vi "rasterScanning.vi"() -> ()   [LabVIEW 2017]
uses:
  <vilib>/rvi/Emulation/niFpgaSctlEmulationGetInTimedLoop.vi
  <vilib>/rvi/Emulation/niFpgaProcessEmulError.vi
  <vilib>/rvi/Emulation/niFpgaGetClockAttributes.vi
  <vilib>/rvi/Emulation/niFpgaEmulationReportErrorSimple.vi
  <vilib>/rvi/eio/common/nirviEmuTemplateMethod_errors.vi
  <vilib>/rvi/Emulation/niFpgaCriticalErrorInLSC.vi
  <vilib>/rvi/interface/RandomDataEmulation/niFpgaRandomDataHandleErrors.vi
  <vilib>/eio/EIONode/EIONode.xnode
  <vilib>/rvi/DataTransferAndStorage/Container/XNode/niFpgaContainer.xnode
  <vilib>/rvi/interface/RandomDataEmulation/nirviRandomDataFpgaReadWriteTemplate.vi
panel:
  in  "y threshold":fxp<+/-,20,5>=0.0050048828125
  in  "x threshold":fxp<+/-,20,5>=0.0050048828125
  out "SettleCheckBuffer":u16=25
  out "a tor buffer":fxp<+,17,1>[](array[numeric])=[1.9999847412109375, 1.9999847412109375, 1.9999847412109375, 1.9999847412109375, 1.9999847412109375, 1.9999847412109375, 1.9999847412109375, 1.9999847412109375, 1.9999847412109375, 1.9999847412109375, 1.9999847412109375, 1.9999847412109375, 1.9999847412109375, 1.9999847412109375, 1.9999847412109375, 1.9999847412109375, 1.9999847412109375, 1.9999847412109375, 1.9999847412109375, 1.9999847412109375, 1.9999847412109375, 1.9999847412109375, 1.9999847412109375, 1.9999847412109375, 1.9999847412109375]
  out "b tor buffer":fxp<+,17,1>[](array[numeric])=[1.9999847412109375, 1.9999847412109375, 1.9999847412109375, 1.9999847412109375, 1.9999847412109375, 1.9999847412109375, 1.9999847412109375, 1.9999847412109375, 1.9999847412109375, 1.9999847412109375, 1.9999847412109375, 1.9999847412109375, 1.9999847412109375, 1.9999847412109375, 1.9999847412109375, 1.9999847412109375, 1.9999847412109375, 1.9999847412109375, 1.9999847412109375, 1.9999847412109375, 1.9999847412109375, 1.9999847412109375, 1.9999847412109375, 1.9999847412109375, 1.9999847412109375]
  in  "Stage Clock (uSec)":fxp<+,32,32>=500.0
  in  "deflection threshold":fxp<+/-,20,5>=0.0050048828125
  in  "z threshold":fxp<+/-,20,5>=0.0050048828125
  out "stageIndicator":u8=1
  in  "Scan Clock (uSec)":fxp<+,32,32>=10.0
  out "increment_y_move":fxp<+/-,55,5>=0.01171875
  out "increment_x_move":fxp<+/-,55,5>=0.01171875
  out "increment_x":fxp<+/-,55,5>=0.01171875
  out "x_pos_final":fxp<+/-,50,5>=0.005859375
  out "y_pos_final":fxp<+/-,50,5>=0.005859375
  in  "ImageToSample":T1={"image size_x"=256, "image size_y"=256, "sample start_x"=0.0, "sample start_y"=0.0, "sample end_x"=3.0, "sample end_y"=3.0}
  out "line counter":u16
  out "end line signal":bool
  in  "pixel segment":u32
  in  "deflection control":T2={"SetPoint (V)"=0.0, "scanning I"=0.03125, "scanning P"=0.0498046875, "Initial I (V)"=0.0, "Upper Limit (V)"=8.0, "Lower Limit (V)"=-8.0}
  out "deflection sensor":fxp<+/-,20,5>=-0.271331787109375
  out "zControlMode":bool
  in  "z control":T3={"SetPoint (V)"=-0.19999980926513672, "I"=0.03125, "P"=0.0498046875, "Initial I (V)"=0.0, "Upper Limit (V)"=8.0, "Lower Limit (V)"=-8.0}
  in  "Z Clock (uSec)":fxp<+,32,32>=10.0
  out "signalToRecord":bool
  out "z output":fxp<+/-,64,29>=-3.5890110712498426
  in  "Sampling Clock (uSec)":fxp<+,32,32>=1500.0
  in  "XY Clock (uSec)":fxp<+,32,32>=50.0
  out "y output":fxp<+/-,64,29>=0.29396580904722214
  out "x output":fxp<+/-,64,29>=0.00029289722442626953
  out "x sensor":fxp<+/-,20,5>
  out "y sensor":fxp<+/-,20,5>=-0.285125732421875
  in  "y control":T2={"SetPoint (V)"=0.0, "scanning I"=0.03125, "scanning P"=0.0498046875, "Initial I (V)"=0.0, "Upper Limit (V)"=8.0, "Lower Limit (V)"=-8.0}
  in  "x control":T2={"SetPoint (V)"=0.0, "scanning I"=0.03125, "scanning P"=0.0498046875, "Initial I (V)"=0.0, "Upper Limit (V)"=8.0, "Lower Limit (V)"=-8.0}
  out "signalToStop":bool
  out "x_pos":fxp<+/-,50,5>=0.005859375
  out "y_pos":fxp<+/-,50,5>=0.005859375
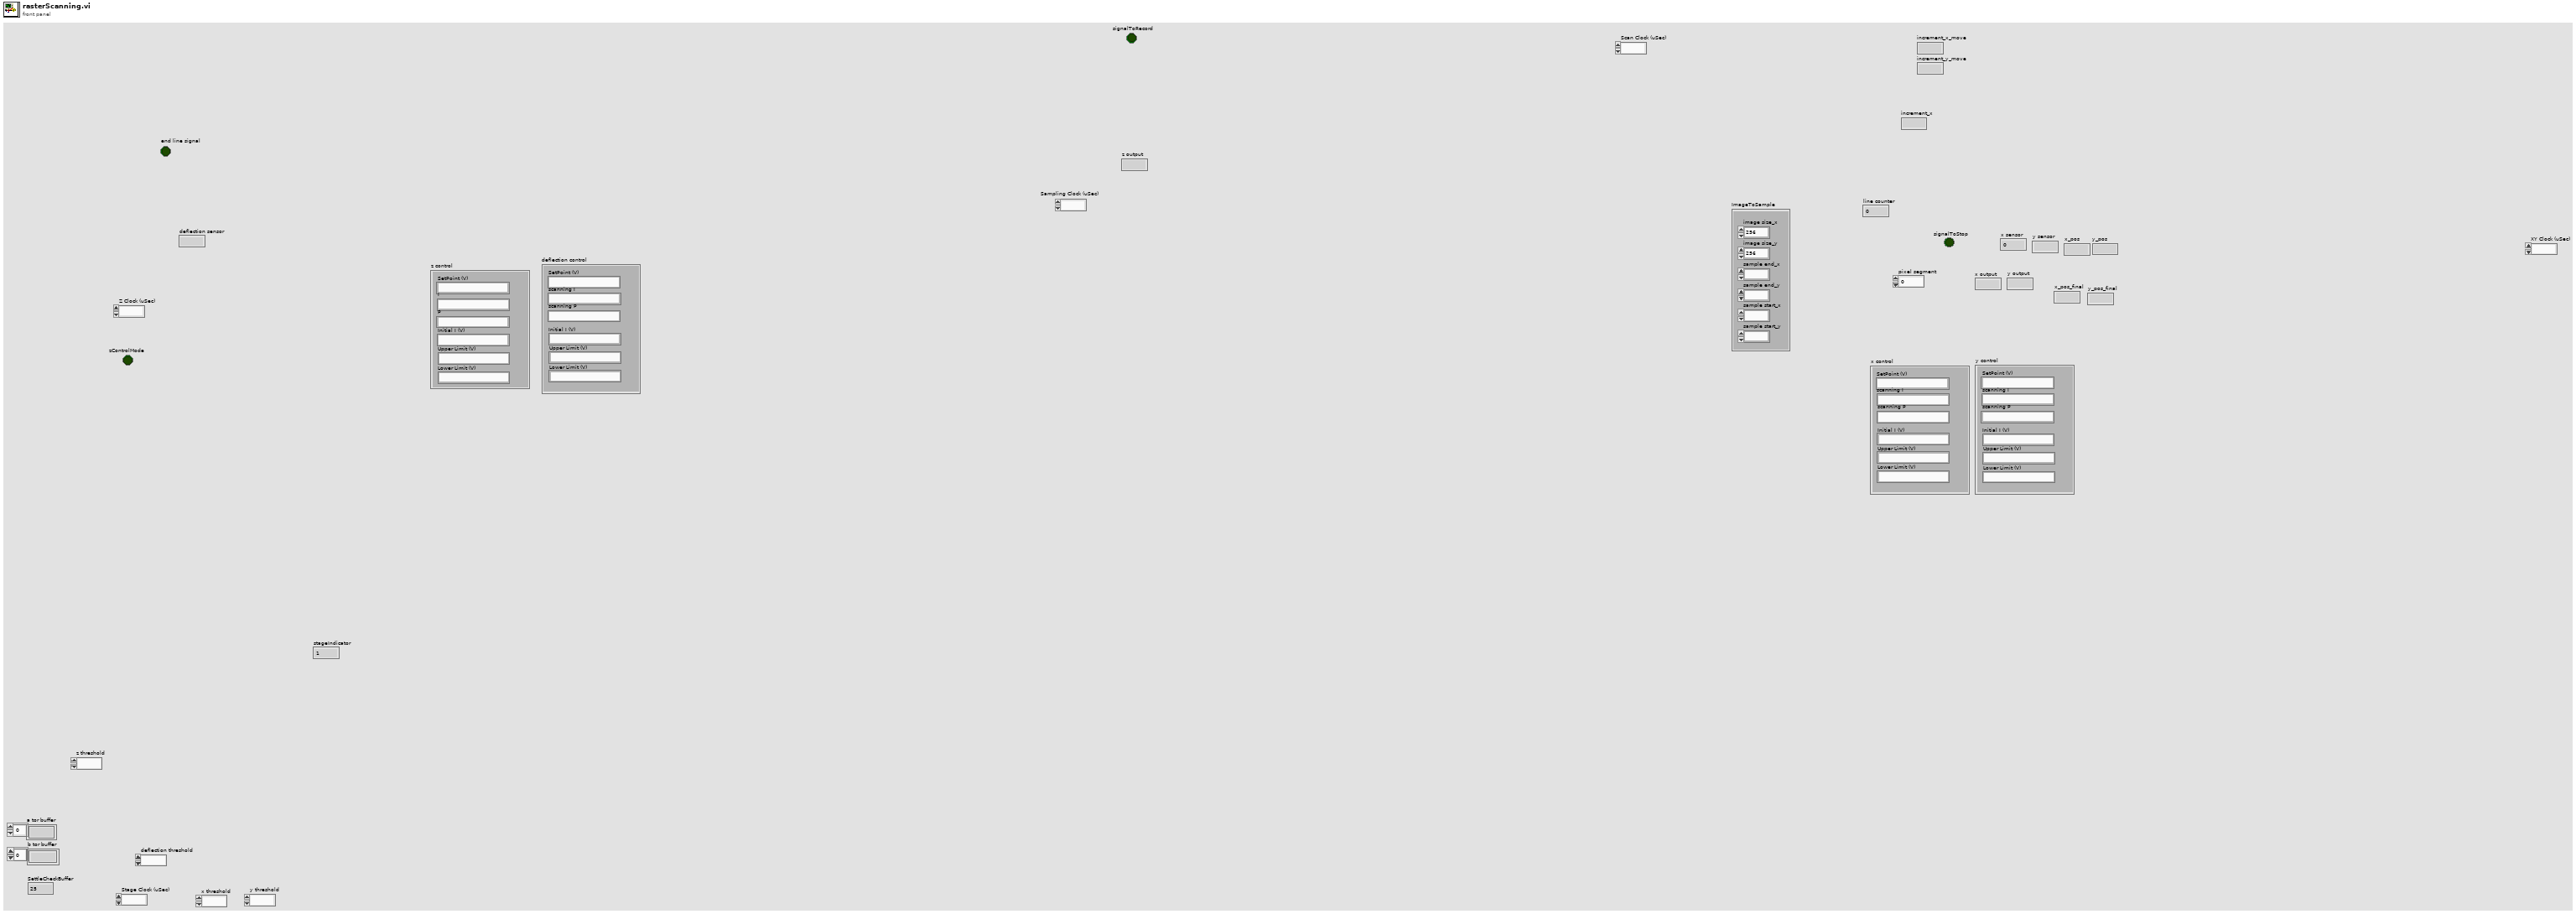
[diagram p1: front panel]
types:
  T1 = cluster{"image size_x":u16, "image size_y":u16, "sample start_x":fxp<+/-,26,5>, "sample start_y":fxp<+/-,26,5>, "sample end_x":fxp<+/-,26,5>, "sample end_y":fxp<+/-,26,5>}
  T2 = cluster{"SetPoint (V)":fxp<+/-,26,5>, "scanning I":fxp<+,21,13>, "scanning P":fxp<+,15,5>, "Initial I (V)":fxp<+/-,10,5>, "Upper Limit (V)":fxp<+/-,26,5>, "Lower Limit (V)":fxp<+/-,26,5>}
  T3 = cluster{"SetPoint (V)":fxp<+/-,26,5>, "I":fxp<+,21,13>, "P":fxp<+,15,5>, "Initial I (V)":fxp<+/-,10,5>, "Upper Limit (V)":fxp<+/-,26,5>, "Lower Limit (V)":fxp<+/-,26,5>}
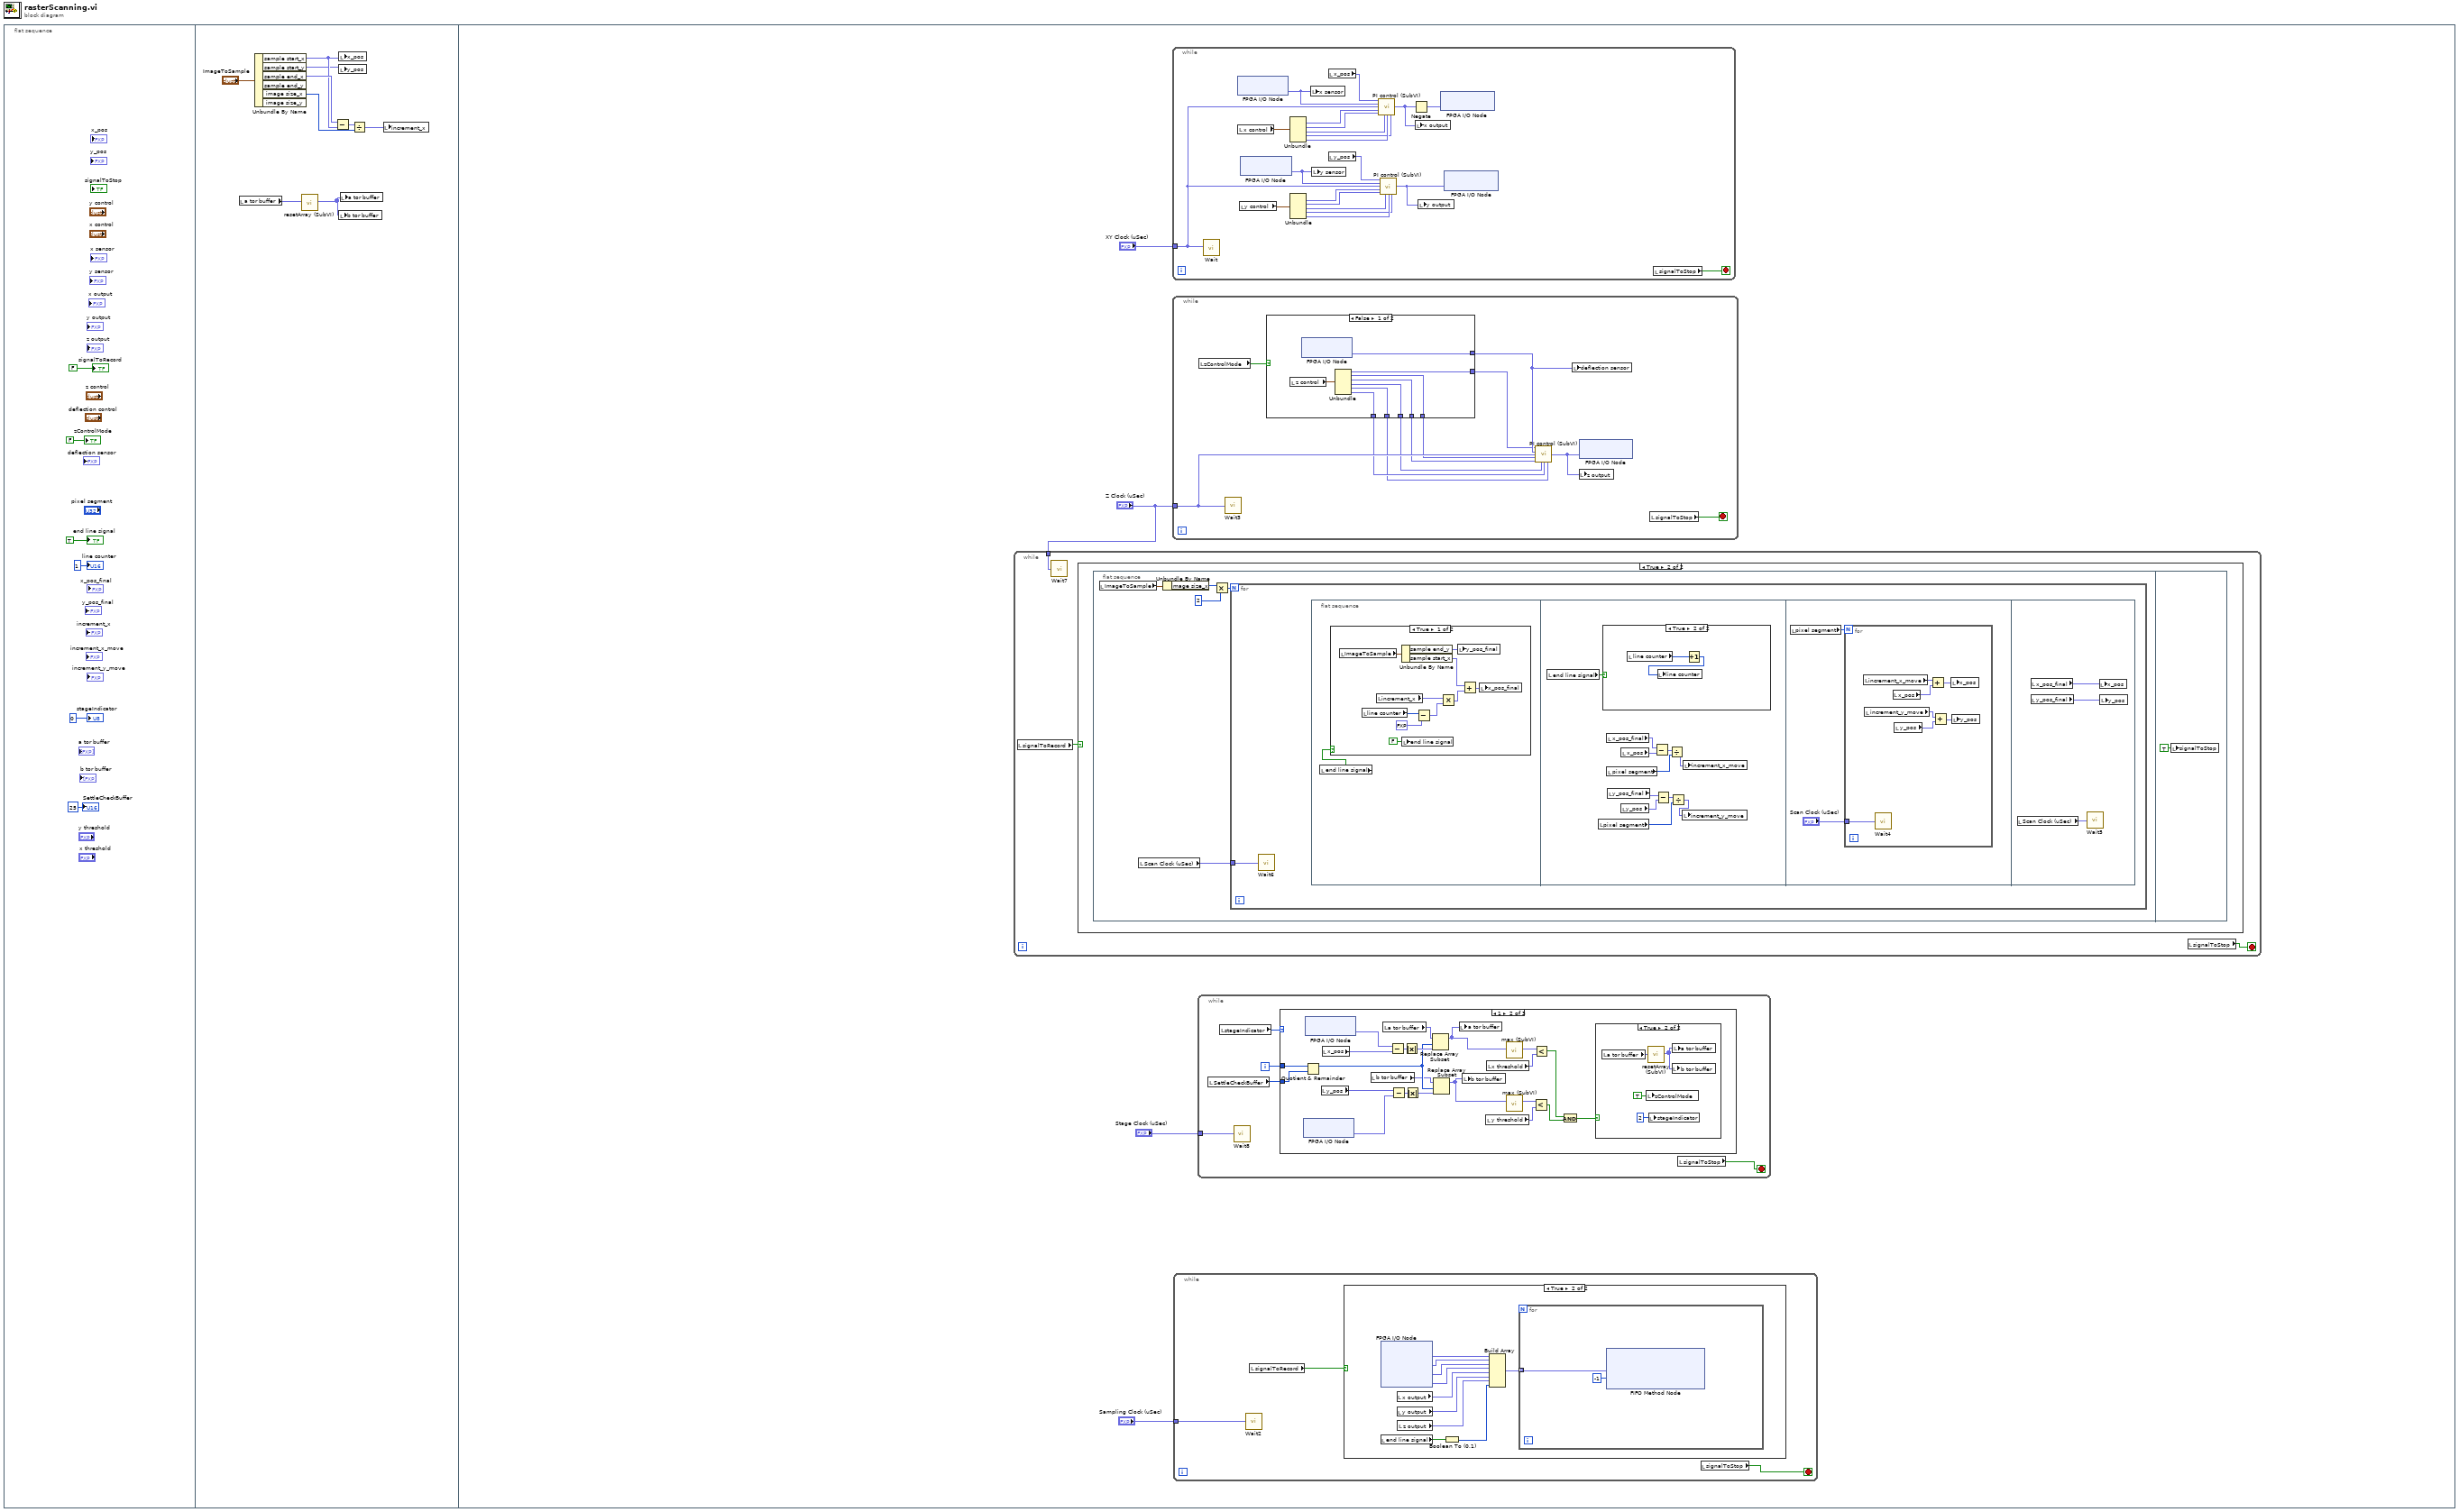
[diagram p0: block diagram]
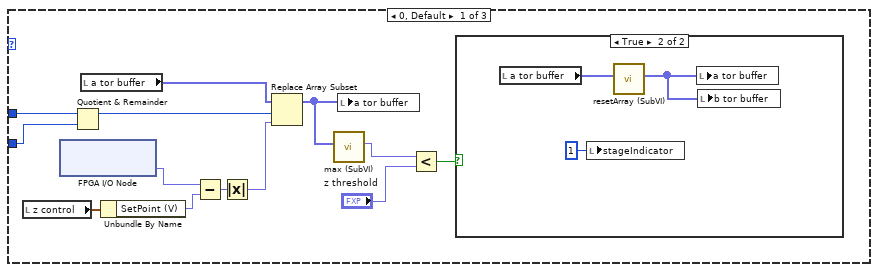
[diagram p2: hidden frame]
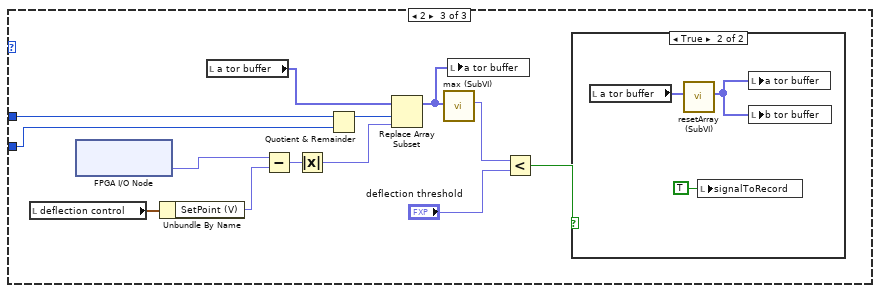
[diagram p5: hidden frame]
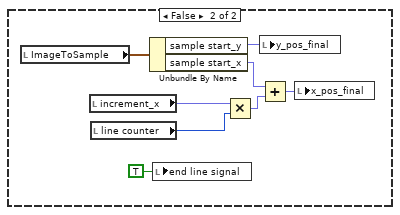
[diagram p8: hidden frame]
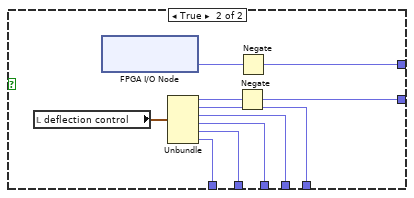
[diagram p10: hidden frame]
diagram:
  n1 = flat-sequence {
    frame #0 {
      "signalToRecord" <- FALSE ("signalToRecord")
      "zControlMode" <- FALSE ("zControlMode")
      "end line signal" <- TRUE ("end line signal")
      "line counter" <- u16 1 ("line counter")
      "stageIndicator" <- u8 0 ("stageIndicator")
      "SettleCheckBuffer" <- u16 25 ("SettleCheckBuffer")
    }
    frame #1 {
      n2 = local read "a tor buffer"() -> (w8:fxp<+,17,1>[])
      n3 = Unbundle By Name("ImageToSample") -> ("sample start_x"=w13:fxp<+/-,26,5>, "sample start_y"=w11:fxp<+/-,26,5>, "sample end_x"=w14:fxp<+/-,26,5>, "image size_x"=w10:u16)  [unwired: 2 out]
      n4 = call "resetArray (SubVI).vi"("a samples in"=w8) -> ("a samples out"=w7:fxp<+/-,64,32>[])  [unwired: 10 in]
      n5 = Subtract(x=w14, y=w13) -> (x-y=w12:fxp<+/-,27,6>)
      n6 = local write "x_pos"(w13) -> ()
      n7 = local write "y_pos"(w11) -> ()
      n8 = local write "b tor buffer"(w7) -> ()
      n9 = local write "a tor buffer"(w7) -> ()
      n10 = Divide(x=w12, y=w10) -> (x/y=w9:fxp<+/-,43,6>)
      n11 = local write "increment_x"(w9) -> ()
    }
    frame #2 {
      n12 = while {
        tunnel: "Z Clock (uSec)" -> [w84]
        stop <- w85 stop-if-true
        n13 = local read "signalToRecord"() -> (w83:bool)
        n14 = call "Wait7"("Count(uSec)"=w84) -> ()  [unwired: 1 out]
        n15 = case shown="True" w83 {
          frame False {
          }
          frame True {
            n16 = flat-sequence {
              frame #0 {
                n17 = local read "ImageToSample"() -> (w90:T1)
                n18 = local read "Scan Clock (uSec)"() -> (w86:fxp<+,32,32>)
                n19 = Unbundle By Name(w90) -> ("image size_x"=w88:u16)
                n20 = Multiply(x=w88, y=u16 2) -> (x*y=w89:u16)
                n21 = for {
                  N: w89 -> [_]
                  tunnel: w86 -> [w91]
                  n22 = call "Wait6"("Count(uSec)"=w91) -> ()  [unwired: 1 out]
                  n23 = flat-sequence {
                    frame #0 {
                      n24 = local read "end line signal"() -> (w92:bool)
                      n25 = case shown="True" w92 {
                        frame True {
                          n26 = local read "ImageToSample"() -> (w102:T1)
                          n27 = local read "line counter"() -> (w98:u16)
                          n28 = local read "increment_x"() -> (w99:fxp<+/-,55,5>)
                          n29 = Unbundle By Name(w102) -> ("sample end_y"=w101:fxp<+/-,26,5>, "sample start_x"=w100:fxp<+/-,26,5>)
                          n30 = local write "end line signal"(FALSE ("end line signal")) -> ()
                          n31 = Subtract(x=w98, y=fxp<+,1,0> 0.5) -> (x-y=w96:fxp<+/-,18,17>)
                          n32 = Multiply(x=w99, y=w96) -> (x*y=w95:fxp<+/-,64,21>)
                          n33 = local write "y_pos_final"(w101) -> ()
                          n34 = Add(x=w100, y=w95) -> (x+y=w94:fxp<+/-,64,22>)
                          n35 = local write "x_pos_final"(w94) -> ()
                        }
                        frame False {
                          n36 = local read "ImageToSample"() -> (w110:T1)
                          n37 = local read "increment_x"() -> (w105:fxp<+/-,55,5>)
                          n38 = local read "line counter"() -> (w104:u16)
                          n39 = Unbundle By Name(w110) -> ("sample start_y"=w109:fxp<+/-,26,5>, "sample start_x"=w108:fxp<+/-,26,5>)
                          n40 = local write "end line signal"(TRUE ("end line signal")) -> ()
                          n41 = Multiply(x=w105, y=w104) -> (x*y=w106:fxp<+/-,64,21>)
                          n42 = local write "y_pos_final"(w109) -> ()
                          n43 = Add(x=w108, y=w106) -> (x+y=w107:fxp<+/-,64,22>)
                          n44 = local write "x_pos_final"(w107) -> ()
                        }
                      }
                    }
                    frame #1 {
                      n45 = local read "end line signal"() -> (w121:bool)
                      n46 = local read "pixel segment"() -> (w119:u32)
                      n47 = case shown="True" w121 {
                        frame False {
                        }
                        frame True {
                          n48 = local read "line counter"() -> (w123:u16)
                          n49 = Increment(x=w123) -> (x+1=w122:u16)
                          n50 = local write "line counter"(w122) -> ()
                        }
                      }
                      n51 = local read "x_pos_final"() -> (w111:fxp<+/-,50,5>)
                      n52 = local read "pixel segment"() -> (w114:u32)
                      n53 = local read "y_pos_final"() -> (w117:fxp<+/-,50,5>)
                      n54 = local read "y_pos"() -> (w118:fxp<+/-,50,5>)
                      n55 = local read "x_pos"() -> (w112:fxp<+/-,50,5>)
                      n56 = Subtract(x=w111, y=w112) -> (x-y=w113:fxp<+/-,51,6>)
                      n57 = Subtract(x=w117, y=w118) -> (x-y=w116:fxp<+/-,51,6>)
                      n58 = Divide(x=w113, y=w114) -> (x/y=w115:fxp<+/-,64,6>)
                      n59 = Divide(x=w116, y=w119) -> (x/y=w120:fxp<+/-,64,6>)
                      n60 = local write "increment_y_move"(w120) -> ()
                      n61 = local write "increment_x_move"(w115) -> ()
                    }
                    frame #2 {
                      n62 = local read "pixel segment"() -> (w125:u32)
                      n63 = for {
                        N: w125 -> [_]
                        tunnel: "Scan Clock (uSec)" -> [w132]
                        n64 = local read "increment_x_move"() -> (w131:fxp<+/-,55,5>)
                        n65 = local read "increment_y_move"() -> (w128:fxp<+/-,55,5>)
                        n66 = call "Wait4"("Count(uSec)"=w132) -> ()  [unwired: 1 out]
                        n67 = local read "x_pos"() -> (w130:fxp<+/-,50,5>)
                        n68 = local read "y_pos"() -> (w127:fxp<+/-,50,5>)
                        n69 = Add(x=w131, y=w130) -> (x+y=w129:fxp<+/-,56,6>)
                        n70 = Add(x=w128, y=w127) -> (x+y=w126:fxp<+/-,56,6>)
                        n71 = local write "x_pos"(w129) -> ()
                        n72 = local write "y_pos"(w126) -> ()
                      }
                    }
                    frame #3 {
                      n73 = local read "Scan Clock (uSec)"() -> (w133:fxp<+,32,32>)
                      n74 = local read "x_pos_final"() -> (w135:fxp<+/-,50,5>)
                      n75 = local read "y_pos_final"() -> (w134:fxp<+/-,50,5>)
                      n76 = call "Wait5"("Count(uSec)"=w133) -> ()  [unwired: 1 out]
                      n77 = local write "x_pos"(w135) -> ()
                      n78 = local write "y_pos"(w134) -> ()
                    }
                  }
                }
              }
              frame #1 {
                n79 = local write "signalToStop"(TRUE ("signalToStop")) -> ()
              }
            }
          }
        }
        n80 = local read "signalToStop"() -> (w85:bool)
      }
      n81 = while {
        tunnel: "XY Clock (uSec)" -> [w187]
        stop <- w201 stop-if-true
        n82 = call "Wait"("Count(uSec)"=w187) -> ()  [unwired: 1 out]
        n83 = xnode "FPGA I/O Node"() -> ("Mod1/AI0"=w198:fxp<+/-,20,5>)  [unwired: 1 in, 1 out]
        n84 = local read "x control"() -> (w200:T2)
        n85 = local read "y control"() -> (w188:T2)
        n86 = xnode "FPGA I/O Node"() -> ("Mod1/AI1"=w189:fxp<+/-,20,5>)  [unwired: 1 in, 1 out]
        n87 = Unbundle(w200) -> ("scanning I"=w197:fxp<+,21,13>, "scanning P"=w196:fxp<+,15,5>, "Initial I (V)"=w195:fxp<+/-,10,5>, "Upper Limit (V)"=w193:fxp<+/-,26,5>, "Lower Limit (V)"=w194:fxp<+/-,26,5>)  [unwired: 1 out]
        n88 = Unbundle(w188) -> ("scanning I"=w186:fxp<+,21,13>, "scanning P"=w185:fxp<+,15,5>, "Initial I (V)"=w184:fxp<+/-,10,5>, "Upper Limit (V)"=w182:fxp<+/-,26,5>, "Lower Limit (V)"=w183:fxp<+/-,26,5>)  [unwired: 1 out]
        n89 = local write "x sensor"(w198) -> ()
        n90 = local write "y sensor"(w189) -> ()
        n91 = local read "x_pos"() -> (w199:fxp<+/-,50,5>)
        n92 = local read "y_pos"() -> (w190:fxp<+/-,50,5>)
        n93 = call "PI control (SubVI).vi"("SetPoint"=w199, "Feedback"=w198, "Clock"=w187, "I"=w197, "P"=w196, "Initial I"=w195, "Lower Limit"=w194, "Upper Limit in"=w193) -> ("Output"=w192:fxp<+/-,20,5>)  [unwired: 7 in]
        n94 = call "PI control (SubVI).vi"("SetPoint"=w190, "Feedback"=w189, "Clock"=w187, "I"=w186, "P"=w185, "Initial I"=w184, "Lower Limit"=w183, "Upper Limit in"=w182) -> ("Output"=w181:fxp<+/-,20,5>)  [unwired: 7 in]
        n95 = Negate(x=w192) -> (-x=w191:fxp<+/-,21,6>)
        n96 = local write "x output"(w192) -> ()
        n97 = local write "y output"(w181) -> ()
        n98 = xnode "FPGA I/O Node"("Mod8/AO0"=w191) -> ()  [unwired: 1 in, 1 out]
        n99 = xnode "FPGA I/O Node"("Mod8/AO1"=w181) -> ()  [unwired: 1 in, 1 out]
        n100 = local read "signalToStop"() -> (w201:bool)
      }
      n101 = while {
        tunnel: "Z Clock (uSec)" -> [w142]
        stop <- w147 stop-if-true
        n102 = local read "zControlMode"() -> (w146:bool)
        n103 = call "Wait3"("Count(uSec)"=w142) -> ()  [unwired: 1 out]
        n104 = case shown="False" w146 {
          tunnel: [w154 w163] -> w144
          tunnel: [w153 w161] -> w143
          tunnel: [w152 w160] -> w141
          tunnel: [w151 w159] -> w140
          tunnel: [w150 w158] -> w139
          tunnel: [w149 w157] -> w138
          tunnel: [w148 w156] -> w137
          frame False {
            n105 = local read "z control"() -> (w155:T3)
            n106 = xnode "FPGA I/O Node"() -> ("Mod1/AI2"=w154:fxp<+/-,20,5>)  [unwired: 1 in, 1 out]
            n107 = Unbundle(w155) -> ("SetPoint (V)"=w153:fxp<+/-,26,5>, "I"=w152:fxp<+,21,13>, "P"=w151:fxp<+,15,5>, "Initial I (V)"=w150:fxp<+/-,10,5>, "Upper Limit (V)"=w148:fxp<+/-,26,5>, "Lower Limit (V)"=w149:fxp<+/-,26,5>)
          }
          frame True {
            n108 = local read "deflection control"() -> (w165:T2)
            n109 = xnode "FPGA I/O Node"() -> ("Mod1/AI3"=w164:fxp<+/-,20,5>)  [unwired: 1 in, 1 out]
            n110 = Unbundle(w165) -> ("SetPoint (V)"=w162:fxp<+/-,26,5>, "scanning I"=w160:fxp<+,21,13>, "scanning P"=w159:fxp<+,15,5>, "Initial I (V)"=w158:fxp<+/-,10,5>, "Upper Limit (V)"=w156:fxp<+/-,26,5>, "Lower Limit (V)"=w157:fxp<+/-,26,5>)
            n111 = Negate(x=w162) -> (-x=w161:fxp<+/-,27,6>)
            n112 = Negate(x=w164) -> (-x=w163:fxp<+/-,21,6>)
          }
        }
        n113 = call "PI control (SubVI).vi"("SetPoint"=w143, "Feedback"=w144, "Clock"=w142, "I"=w141, "P"=w140, "Initial I"=w139, "Lower Limit"=w138, "Upper Limit in"=w137) -> ("Output"=w145:fxp<+/-,20,5>)  [unwired: 7 in]
        n114 = local write "deflection sensor"(w144) -> ()
        n115 = xnode "FPGA I/O Node"("Mod8/AO2"=w145) -> ()  [unwired: 1 in, 1 out]
        n116 = local write "z output"(w145) -> ()
        n117 = local read "signalToStop"() -> (w147:bool)
      }
      n118 = while {
        tunnel: "Sampling Clock (uSec)" -> [w168]
        stop <- w167 stop-if-true
        n119 = call "Wait2"("Count(uSec)"=w168) -> ()  [unwired: 1 out]
        n120 = local read "signalToRecord"() -> (w166:bool)
        n121 = case shown="True" w166 {
          frame False {
          }
          frame True {
            n122 = local read "end line signal"() -> (w170:bool)
            n123 = xnode "FPGA I/O Node"() -> ("Mod1/AI0"=w178:fxp<+/-,20,5>, "Mod1/AI1"=w177:fxp<+/-,20,5>, "Mod1/AI2"=w176:fxp<+/-,20,5>, "Mod1/AI3"=w175:fxp<+/-,20,5>)  [unwired: 4 in, 4 out]
            n124 = local read "x output"() -> (w174:fxp<+/-,64,29>)
            n125 = local read "y output"() -> (w173:fxp<+/-,64,29>)
            n126 = local read "z output"() -> (w172:fxp<+/-,64,29>)
            n127 = Boolean To (0,1)(Boolean=w170) -> (0, 1=w169:i16)
            n128 = Build Array(w178, w177, w176, w175, w174, w173, w172, w169) -> (w171:fxp<+/-,64,29>[])
            n129 = for {
              tunnel: w171 -> [w180] mode=indexing
              n130 = xnode ("FIFO Method Node")("Element"=w180, "Timeout"=-1) -> ()  [unwired: 1 in, 2 out]
            }
          }
        }
        n131 = local read "signalToStop"() -> (w167:bool)
      }
      n132 = while {
        tunnel: "Stage Clock (uSec)" -> [w24]
        i -> [w22]
        stop <- w20 stop-if-true
        n133 = local read "SettleCheckBuffer"() -> (w21:u16)
        n134 = local read "stageIndicator"() -> (w23:u8)
        n135 = call "Wait8"("Count(uSec)"=w24) -> ()  [unwired: 1 out]
        n136 = case shown="1" w23 {
          tunnel: w22 -> [w37 w62 w79]
          tunnel: w21 -> [w36 w61 w78]
          frame 0, Default {
            n137 = local read "z control"() -> (w30:T3)
            n138 = xnode "FPGA I/O Node"() -> ("Mod1/AI2"=w32:fxp<+/-,20,5>)  [unwired: 1 in, 1 out]
            n139 = Quotient & Remainder(x=w37, y=w36) -> (x-y*floor(x/y)=w35:i32)  [unwired: 1 out]
            n140 = local read "a tor buffer"() -> (w31:fxp<+,17,1>[])
            n141 = Unbundle By Name(w30) -> ("SetPoint (V)"=w29:fxp<+/-,26,5>)
            n142 = Subtract(x=w32, y=w29) -> (x-y=w34:fxp<+/-,27,6>)
            n143 = Absolute Value(x=w34) -> (abs(x)=w33:fxp<+,26,5>)
            n144 = Replace Array Subset(array=w31, new element=w33, index=w35) -> (w28:fxp<+,17,1>[])
            n145 = call "max (SubVI).vi"("initialized array"=w28) -> ("y"=w27:fxp<+/-,64,32>)  [unwired: 10 in]
            n146 = local write "a tor buffer"(w28) -> ()
            n147 = Less?(x=w27, y="z threshold") -> (x < y?=w25:bool)
            n148 = case shown="True" w25 {
              frame False {
              }
              frame True {
                n149 = local read "a tor buffer"() -> (w40:fxp<+,17,1>[])
                n150 = local write "stageIndicator"(u8 1 ("stageIndicator")) -> ()
                n151 = call "resetArray (SubVI).vi"("a samples in"=w40) -> ("a samples out"=w39:fxp<+/-,64,32>[])  [unwired: 10 in]
                n152 = local write "a tor buffer"(w39) -> ()
                n153 = local write "b tor buffer"(w39) -> ()
              }
            }
          }
          frame 1 {
            n154 = xnode "FPGA I/O Node"() -> ("Mod1/AI1"=w43:fxp<+/-,20,5>)  [unwired: 1 in, 1 out]
            n155 = Quotient & Remainder(x=w62, y=w61) -> (x-y*floor(x/y)=w53:i32)  [unwired: 1 out]
            n156 = xnode "FPGA I/O Node"() -> ("Mod1/AI0"=w44:fxp<+/-,20,5>)  [unwired: 1 in, 1 out]
            n157 = local read "y_pos"() -> (w41:fxp<+/-,50,5>)
            n158 = local read "x_pos"() -> (w42:fxp<+/-,50,5>)
            n159 = local read "b tor buffer"() -> (w51:fxp<+,17,1>[])
            n160 = local read "a tor buffer"() -> (w52:fxp<+,17,1>[])
            n161 = Subtract(x=w44, y=w42) -> (x-y=w57:fxp<+/-,51,6>)
            n162 = Subtract(x=w41, y=w43) -> (x-y=w55:fxp<+/-,51,6>)
            n163 = Absolute Value(x=w57) -> (abs(x)=w56:fxp<+,50,5>)
            n164 = Absolute Value(x=w55) -> (abs(x)=w54:fxp<+,50,5>)
            n165 = Replace Array Subset(array=w52, new element=w56, index=w53) -> (w50:fxp<+,17,1>[])
            n166 = Replace Array Subset(array=w51, new element=w54, index=w53) -> (w49:fxp<+,17,1>[])
            n167 = local write "a tor buffer"(w50) -> ()
            n168 = local write "b tor buffer"(w49) -> ()
            n169 = local read "y threshold"() -> (w45:fxp<+/-,20,5>)
            n170 = local read "x threshold"() -> (w47:fxp<+/-,20,5>)
            n171 = call "max (SubVI).vi"("initialized array"=w50) -> ("y"=w48:fxp<+/-,64,32>)  [unwired: 10 in]
            n172 = call "max (SubVI).vi"("initialized array"=w49) -> ("y"=w46:fxp<+/-,64,32>)  [unwired: 10 in]
            n173 = Less?(x=w46, y=w45) -> (x < y?=w59:bool)
            n174 = Less?(x=w48, y=w47) -> (x < y?=w60:bool)
            n175 = And(x=w60, y=w59) -> (x .and. y?=w58:bool)
            n176 = case shown="True" w58 {
              frame False {
              }
              frame True {
                n177 = local read "a tor buffer"() -> (w65:fxp<+,17,1>[])
                n178 = local write "zControlMode"(TRUE ("zControlMode")) -> ()
                n179 = call "resetArray (SubVI).vi"("a samples in"=w65) -> ("a samples out"=w64:fxp<+/-,64,32>[])  [unwired: 10 in]
                n180 = local write "stageIndicator"(u8 2 ("stageIndicator")) -> ()
                n181 = local write "b tor buffer"(w64) -> ()
                n182 = local write "a tor buffer"(w64) -> ()
              }
            }
          }
          frame 2 {
            n183 = local read "deflection control"() -> (w75:T2)
            n184 = xnode "FPGA I/O Node"() -> ("Mod1/AI3"=w73:fxp<+/-,20,5>)  [unwired: 1 in, 1 out]
            n185 = Unbundle By Name(w75) -> ("SetPoint (V)"=w74:fxp<+/-,26,5>)
            n186 = local read "a tor buffer"() -> (w69:fxp<+,17,1>[])
            n187 = Subtract(x=w73, y=w74) -> (x-y=w77:fxp<+/-,27,6>)
            n188 = Absolute Value(x=w77) -> (abs(x)=w72:fxp<+,26,5>)
            n189 = Quotient & Remainder(x=w79, y=w78) -> (x-y*floor(x/y)=w76:i32)  [unwired: 1 out]
            n190 = Replace Array Subset(array=w69, new element=w72, index=w76) -> (w68:fxp<+,17,1>[])
            n191 = call "max (SubVI).vi"("initialized array"=w68) -> ("y"=w71:fxp<+/-,64,32>)  [unwired: 10 in]
            n192 = local write "a tor buffer"(w68) -> ()
            n193 = Less?(x=w71, y="deflection threshold") -> (x < y?=w67:bool)
            n194 = case shown="True" w67 {
              frame False {
              }
              frame True {
                n195 = local read "a tor buffer"() -> (w82:fxp<+,17,1>[])
                n196 = call "resetArray (SubVI).vi"("a samples in"=w82) -> ("a samples out"=w81:fxp<+/-,64,32>[])  [unwired: 10 in]
                n197 = local write "signalToRecord"(TRUE ("signalToRecord")) -> ()
                n198 = local write "a tor buffer"(w81) -> ()
                n199 = local write "b tor buffer"(w81) -> ()
              }
            }
          }
        }
        n200 = local read "signalToStop"() -> (w20:bool)
      }
    }
  }
